vi "Get Resource Type.vi"(4 "PWM in":refnum<class "PWM.lvclass">) -> (7 "Resource Type":string)   [LabVIEW 2020, in "CTI.lvlib" / "PWM.lvclass"]
uses:
  PWM.lvclass
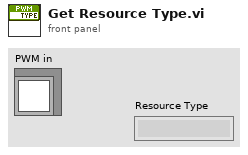
[diagram p1: front panel]
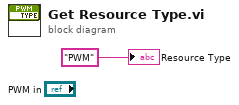
[diagram p0: block diagram]
diagram:
  "Resource Type" <- "PWM" ("Resource Type")
